vi "Scan Double.vi"(8 "error in (no error)":errorcluster, 11 "Scan Driver in":refnum<class "Scan Driver.lvclass">) -> (0 "error out":errorcluster, 2 "Again?":bool, 3 "Scan Driver out":refnum<class "Scan Driver.lvclass">)   [LabVIEW 2012, in "Scan Driver.lvclass"]
doc: "Main method for Scan Driver. Scan over the given Scanner, read data points from the given Readable, generate an onscreen graph, and write a data file."
uses:
  Scan Driver.lvclass
  File IO/File IO.lvclass
  Global/File Locations.vi
  Global/Flags.vi
  Global/Misc.vi
  Scan Graph.ctl
  Scanners/Scanner/Scanner.lvclass
  Readers/Reader/Reader.lvclass
  Scanners/Double Scanner/Double Scanner.lvclass
  Instruments/Utility Classes/Readable/X.ctl
  Instruments/Utility Classes/Readable/Readable.lvclass
panel:
  out "Data Monitor 2D":T2(array[cluster])
  out "?":string
  out "progress":string
  out "Time Estimate":string
  out "date":timestamp
  out "timedisp":string
  in  "log?":bool
  out "cpshigh":dbl caption="CPS High"
  in  "restart":bool
  out "busybar":bool[](array[boolean])
  out "done?":bool caption="Done"
  in  "Exit":bool
  in  "stop":bool
  in  "?":bool
  out "Primary Graph":T3(graph) caption="cpsgraph"
  out "time":dbl
  out "Secondary Graph":T3(graph)
  # "Log"
  # "Linear"
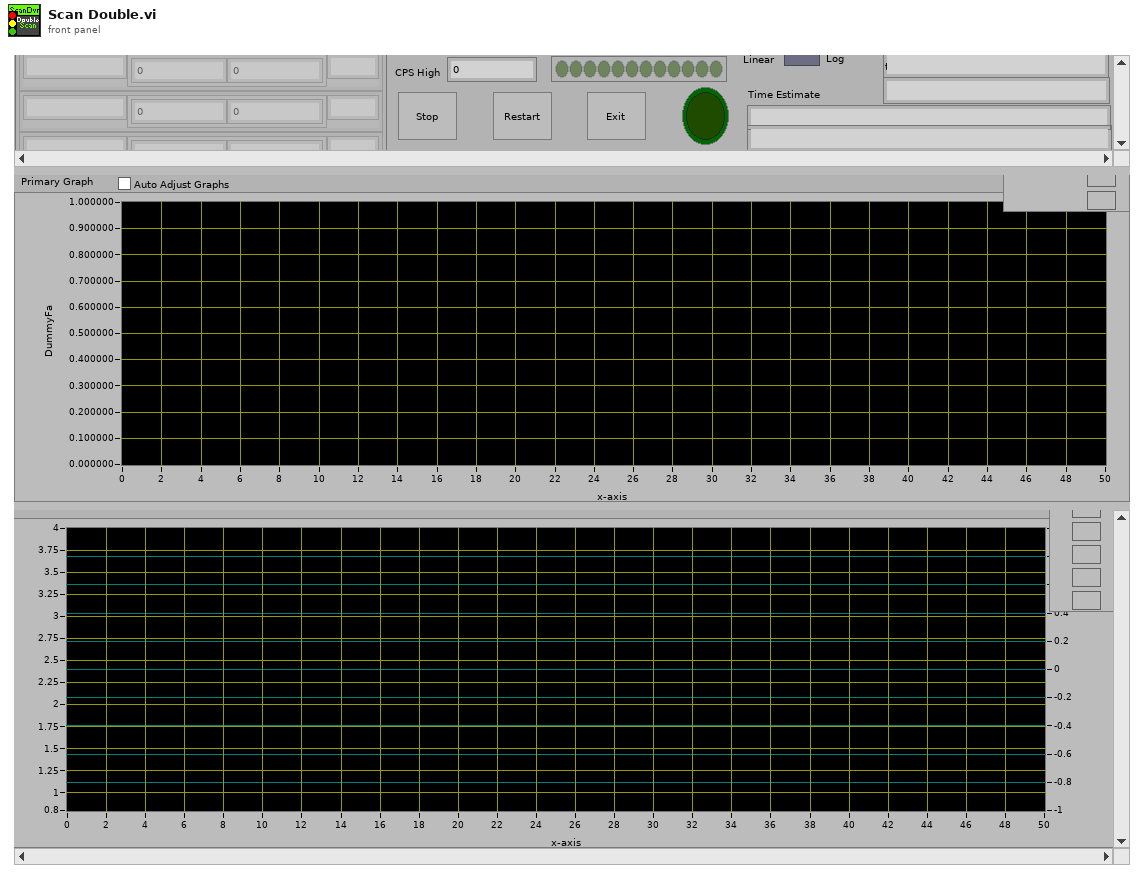
[diagram p1: front panel]
types:
  T1 = typedef "Readable.lvclass/X.ctl" = dbl
  T2 = cluster{"Name":string, "Array":T1[], "Unit":string}[]
  T3 = typedef "Scan Driver.lvclass/Scan Graph.ctl" = cluster{"point array":cluster{"x":dbl, "y":dbl}[]}[]
  T4 = typedef "Scanner.lvclass/Range.ctl" = cluster{"xi":dbl, "xf":dbl, "dx":dbl, "Return to...?":bool, "Return to":dbl}
  T5 = typedef "Readable.lvclass/Data Channels.ctl" = T6[]
  T6 = typedef "Readable.lvclass/Data Channel.ctl" = cluster{"Name":string, "Data Point":T7, "Unit":string}
  T7 = typedef "Readable.lvclass/Data Point.ctl" = cluster{"t":T8, "x":T1}
  T8 = typedef "Readable.lvclass/Time.ctl" = timestamp
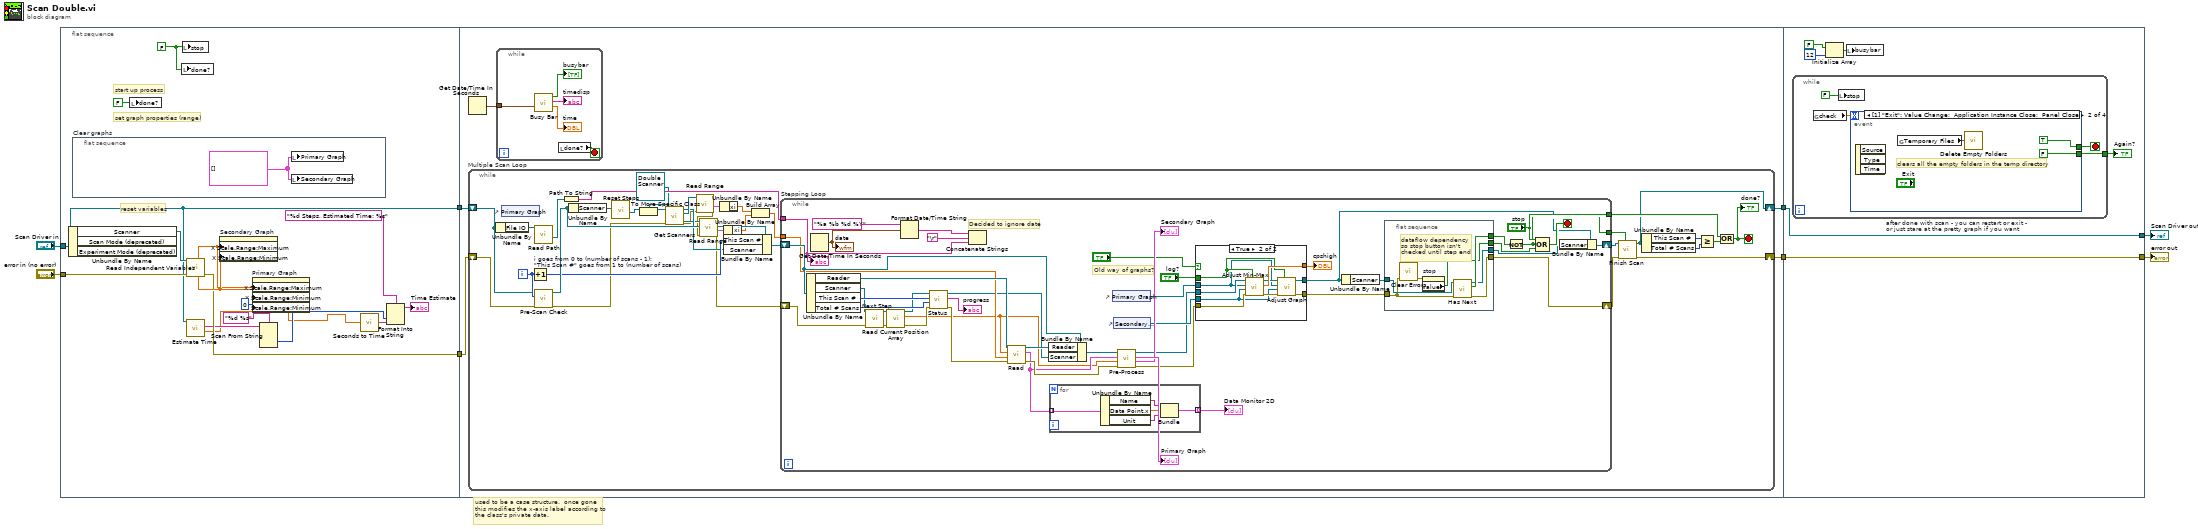
[diagram p0: block diagram]
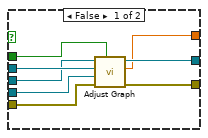
[diagram p2: hidden frame]
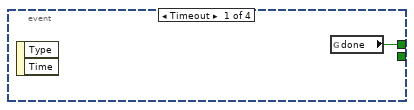
[diagram p3: hidden frame]
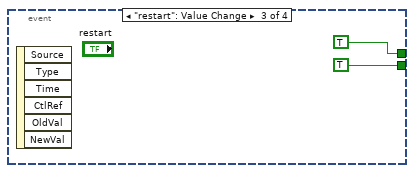
[diagram p4: hidden frame]
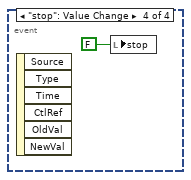
[diagram p5: hidden frame]
diagram:
  # "used to be a case structure.  once gone\nthis modifies the x-axis label according to\nthe class's private data."
  n1 = flat-sequence {
    tunnel: [w17] -> w4
    tunnel: [w21] -> w3
    tunnel: "error in (no error)" -> [w20]
    tunnel: "Scan Driver in" -> [w17]
    tunnel: w4 -> [w29]
    tunnel: [w28] -> w2
    tunnel: w3 -> [w27]
    tunnel: [w26] -> w1
    tunnel: [w147] -> w8
    tunnel: [w146] -> w5
    tunnel: w2 -> [w147]
    tunnel: w1 -> [w146]
    frame #0 {
      w19 = FALSE
      # "reset variables"
      # "start up process"
      # "set graph properties (range)"
      n2 = Unbundle By Name(w17) -> ("Scanner"=w18:refnum<class "Scanner.lvclass">)  [unwired: 2 out]
      n3 = flat-sequence "Clear graphs" {
        frame #0 {
          w25 = T3 []
          n4 = local write "Primary Graph"(w25) -> ()
          n5 = local write "Secondary Graph"(w25) -> ()
        }
      }
      n6 = local write "done?"(FALSE) -> ()
      n7 = local write "done?"(w19) -> ()
      n8 = local write "stop"(w19) -> ()
      n9 = call-dynamic "Read Independent Variables.vi"("error in (no error)"=w20, "Scanner.lvclass in"=w18) -> ("error out"=w21:errorcluster, "min value"=w24:dbl, "max value"=w23:dbl)  [unwired: 7 out]
      n10 = call "Estimate Time.vi"("Scan Driver in"=w17) -> ("Seconds"=w9:dbl[unit], "Time Estimate"=w15:string)  [unwired: 1 in, 8 out]
      n11 = property on="Secondary Graph" class="XYGraph (strict)"("X Scale.Range:Maximum"=w23, "X Scale.Range:Minimum"=w24) -> ()  [unwired: 2 in, 2 out]
      n12 = property on="Primary Graph" class="XYGraph (strict)"("X Scale.Range:Maximum"=w23, "X Scale.Range:Minimum"=w24, "Y Scale.Range:Minimum"=0) -> ()  [unwired: 2 in, 2 out]
      n13 = Scan From String(format string="%d %s", input string=w15) -> (output 1=w12:i32)  [unwired: 5 in, 3 out]
      n14 = call "Seconds to Time.vi"("Seconds"=w9) -> ("Time"=w11:string)
      n15 = Format Into String(format string="%d Steps, Estimated Time: %s", w12, w11) -> (resulting string=→"Time Estimate":string)  [unwired: 2 in, 1 out]
    }
    frame #1 {
      n16 = Get Date/Time In Seconds() -> (seconds since 1Jan1904=w30:timestamp)
      n17 = while "Multiple Scan Loop" {
        shift-right: [w61] -> w28
        shift-left: w29 -> [w54]
        shift-right: [w64] -> w26
        shift-left: w27 -> [w60]
        i -> [w55]
        stop <- w68 stop-if-true
        n18 = Unbundle By Name(w54) -> ("File IO"=w53:refnum<class "File IO.lvclass">)
        n19 = control-ref of="Primary Graph"() -> ()  [unwired: 1 out]
        n20 = Increment "i goes from 0 to (number of scans - 1);\n\"This Scan #\" goes from 1 to (number of scans)"(x=w55) -> (x+1=w56:i32)
        n21 = call-dynamic "Read Path.vi"("File IO.lvclass in"=w53) -> ("File Path"=w52:path)  [unwired: 6 in, 4 out]
        n22 = call "Pre-Scan Check.vi"("error in (no error)"=w60, "Current scan #"=w55, "Scan Driver in"=w54) -> ("error out"=w39:errorcluster, "Scan Driver out"=w57:refnum<class "Scan Driver.lvclass">)  [unwired: 2 in, 5 out]
        n23 = Path To String(path=w52) -> (string=w51:string)
        n24 = Unbundle By Name(w57) -> ("Scanner"=w59:refnum<class "Scanner.lvclass">)
        n25 = call "Reset Steps.vi"("Scanner.lvclass"=w59) -> ("Scanner.lvclass"=w47:refnum<class "Scanner.lvclass">)  [unwired: 10 in]
        n26 = To More Specific Class(target class=refnum<class "Double Scanner.lvclass"> refnum ("Double Scanner.lvclass"), reference=w47) -> (specific class reference=w46:refnum<class "Double Scanner.lvclass">)  [unwired: 1 in, 1 out]
        n27 = call-dynamic "Get Scanners.vi"("error in (no error)"=w39, "Double Scanner in"=w46) -> ("error out"=w38:errorcluster, "Scanner 2 out"=w42:refnum<class "Scanner.lvclass">, "Scanner 1 out"=w45:refnum<class "Scanner.lvclass">, "Double Scanner out"=w44:refnum<class "Double Scanner.lvclass">)  [unwired: 6 in]
        n28 = call-dynamic "Read Range.vi"("error in (no error)"=w38, "Scanner.lvclass in"=w45) -> ("error out"=w37:errorcluster, "Range"=w50:T4)  [unwired: 8 out]
        n29 = call-dynamic "Read Range.vi"("error in (no error)"=w37, "Scanner.lvclass in"=w42) -> ("error out"=w36:errorcluster, "Range"=w43:T4)  [unwired: 8 out]
        n30 = Unbundle By Name(w50) -> ("xi"=w40:dbl)
        n31 = Unbundle By Name(w43) -> ("xi"=w41:dbl)
        n32 = Bundle By Name(cluster=w57, "This Scan #"=w56, "Scanner"=w44) -> (w58:refnum<class "Scan Driver.lvclass">)
        n33 = Build Array(w40, w41) -> (w49:dbl[])
        n34 = while "Stepping Loop" {
          tunnel: ["stop"] -> w70
          shift-right: [w101] -> w65
          shift-left: w58 -> [w98]
          shift-right: [w104] -> w66
          shift-left: w36 -> [w100]
          tunnel: [w107] -> w63
          tunnel: w49 -> [w95]
          tunnel: w51 -> [w77]
          stop <- w115 stop-if-true
          # "Old way of graphs?"
          # "Decided to ignore date"
          n35 = Unbundle By Name(w98) -> ("Reader"=w97:refnum<class "Reader.lvclass">, "Scanner"=w99:refnum<class "Scanner.lvclass">, "This Scan #"=w106:u32, "Total # Scans"=w109:u32)
          n36 = Get Date/Time In Seconds() -> (seconds since 1Jan1904=w91:timestamp)
          "date" <- w91
          n37 = call-dynamic "Next Step.vi"("error in (no error)"=w100, "Scanner in"=w99) -> ("error out"=w74:errorcluster, "Scanner out"=w75:refnum<class "Scanner.lvclass">)  [unwired: 8 out]
          n38 = call-dynamic "Read Current Position Array.vi"("error in (no error)"=w74, "Scanner in"=w75) -> ("error out"=w73:errorcluster, "Position array"=w72:dbl[], "Scanner out"=w71:refnum<class "Scanner.lvclass">)  [unwired: 7 in]
          n39 = Format Date/Time String(time format string (%c)="%a %b %d %Y", seconds (now)=w91) -> (date/time string=w89:string)  [unwired: 1 in]
          n40 = call-dynamic "Status.vi"("error in (no error)"=w73, "totalscans"=w109, "scan#"=w106, "Scanner.lvclass in"=w71) -> ("error out"=w96:errorcluster, "scanprogress"=→"progress":string, "Scanner.lvclass out"=w87:refnum<class "Scanner.lvclass">)  [unwired: 5 out]
          n41 = Concatenate Strings(w89, "\r", w77) -> ()  [unwired: 1 out]
          n42 = call-dynamic "Read.vi"("error in (no error)"=w96, "Starting independent variables"=w95, "Current independent variables"=w72, "Reader in"=w97) -> ("error out"=w111:errorcluster, "Data Channels"=w93:T5, "Reader out"=w94:refnum<class "Reader.lvclass">)  [unwired: 5 out]
          n43 = Bundle By Name(cluster=w98, "Reader"=w94, "Scanner"=w87) -> (w110:refnum<class "Scan Driver.lvclass">)
          n44 = for {
            tunnel: w93 -> [w145] mode=indexing
            tunnel: [w141] -> w76 mode=indexing
            n45 = Unbundle By Name(w145) -> ("Name"=w142:string, "Data Point.x"=w143:T1, "Unit"=w144:string)
            n46 = Bundle("Name"=w142, "x"=w143, "Unit"=w144) -> (w141:cluster{"Name":string, "x":T1, "Unit":string})  [unwired: 1 in]
          }
          "Data Monitor 2D" <- w76
          n47 = control-ref of="Primary Graph"() -> (w86:refnum<vi>)
          n48 = control-ref of="Secondary Graph"() -> (w85:refnum<vi>)
          n49 = call "Pre-Process.vi"("error in"=w111, "Actual X Positions"=w72, "New Data Points"=w93, "Scan Driver.lvclass in"=w110) -> ("error out"=w83:errorcluster, "Secondary Graph"=→"Secondary Graph":T3, "Primary Graph"=→"Primary Graph":T3, "Scan Driver.lvclass out"=w84:refnum<class "Scan Driver.lvclass">)  [unwired: 3 in, 1 out]
          n50 = case shown="True" "?" {
            tunnel: w86 -> [w123 w125]
            tunnel: w85 -> [w122 w124]
            tunnel: w84 -> [w121 w133]
            tunnel: w83 -> [w120 w132]
            tunnel: [w116 w129] -> w82
            tunnel: [w118 w130] -> w81
            tunnel: [w117 w131] -> w80
            tunnel: "log?" -> [w119 w126]
            frame False {
              n51 = call "Adjust Graph.vi"("log?"=w119, "error in (no error)"=w120, "Secondary Graph"=w122, "Primary Graph"=w123, "Scan Driver.lvclass"=w121) -> ("error out"=w116:errorcluster, "High"=w117:dbl, "Scan Driver.lvclass out"=w118:refnum<class "Scan Driver.lvclass">)  [unwired: 4 in]
            }
            frame True {
              n52 = call "Adjust Min-Max.vi"("log?"=w126, "error in (no error)"=w132, "Secondary Graph"=w124, "Primary Graph"=w125, "Scan Driver.lvclass"=w133) -> ("error out"=w128:errorcluster, "High"=w131:dbl, "Scan Driver.lvclass out"=w127:refnum<class "Scan Driver.lvclass">)  [unwired: 3 in, 1 out]
              n53 = call "Adjust Graph.vi"("log?"=w126, "error in (no error)"=w128, "Secondary Graph"=w124, "Primary Graph"=w125, "Scan Driver.lvclass"=w127) -> ("error out"=w129:errorcluster, "Scan Driver.lvclass out"=w130:refnum<class "Scan Driver.lvclass">)  [unwired: 4 in, 1 out]
            }
          }
          "cpshigh" <- w80
          n54 = Unbundle By Name(w81) -> ("Scanner"=w103:refnum<class "Scanner.lvclass">)
          n55 = flat-sequence {
            tunnel: [w140] -> w105
            tunnel: w82 -> [w135]
            tunnel: [w139] -> w104
            tunnel: w103 -> [w138]
            tunnel: [w137] -> w102
            tunnel: [w134] -> w92
            frame #0 {
              # "dataflow dependency\nso stop button isn't\nchecked until step end"
              n56 = call <vilib>:"Clear Errors.vi"("error in (no error)"=w135) -> ("error out"=w136:errorcluster)  [unwired: 6 in]
              n57 = property on="stop" class="Bool (strict)"(error in=w136) -> ("Value"=w134:bool)  [unwired: 1 in, 2 out]
              n58 = call-dynamic "Has Next.vi"("error in (no error)"=w135, "Scanner.lvclass in"=w138) -> ("error out"=w139:errorcluster, "Again?"=w140:bool, "Scanner.lvclass out"=w137:refnum<class "Scanner.lvclass">)  [unwired: 7 out]
            }
          }
          n59 = Not(x=w105) -> (.not. x?=w107:bool)
          n60 = Compound Arithmetic op=OR("stop", w107, w92) -> (w115:bool)
          n61 = Bundle By Name(cluster=w81, "Scanner"=w102) -> (w101:refnum<class "Scan Driver.lvclass">)
          "?" <- w77
        }
        n62 = call "Finish Scan.vi"("Scan finished successfully?"=w63, "error in"=w66, "Scan Driver.lvclass in"=w65) -> ("error out"=w64:errorcluster, "Scan Driver.lvclass out"=w61:refnum<class "Scan Driver.lvclass">)  [unwired: 2 in, 5 out]
        n63 = Unbundle By Name(w61) -> ("This Scan #"=w62:u32, "Total # Scans"=w67:u32)
        n64 = Greater Or Equal?(x=w62, y=w67) -> (x >= y?=w69:bool)
        n65 = Compound Arithmetic op=OR(w70, w69) -> (w68:bool)
        "done?" <- w68
      }
      n66 = while {
        tunnel: w30 -> [w34]
        stop <- w33 stop-if-true
        n67 = call "Busy Bar.vi"("basetime"=w34) -> ("Elapsed Seconds"=→"time":dbl, "Time"=→"timedisp":string, "Busy Bar"=→"busybar":bool[])  [unwired: 1 in, 7 out]
        n68 = local read "done?"() -> (w33:bool)
      }
    }
    frame #2 {
      n69 = while "after done with scan - you can restart or exit - or just stare at the pretty graph if you want" {
        tunnel: [w153] -> w148
        stop <- w152 stop-if-true
        n70 = global read "Misc.vi" "check"() -> (w154:dbl)
        n71 = local write "stop"(FALSE ("stop")) -> ()
        n72 = event shown="[1] \"Exit\": Value Change;  Application Instance Close;  Panel Close" {
          selector: _ -> [_ _ _ _]
          dyn-events: _ -> [_ _ _ _]
          timeout: w154 -> [_ _ _ _]
          tunnel: [w156 TRUE TRUE ("done") _] -> w152
          tunnel: [_ FALSE TRUE ("done") _] -> w153
          event Timeout {
            n73 = event-data() -> ()  [unwired: 3 out]
            n74 = global read "Flags.vi" "done"() -> (w156:bool)
          }
          event "Exit": Value Change; Application Instance Close; Panel Close {
            # "clears all the empty folders in the temp directory"
            n75 = event-data() -> ()  [unwired: 4 out]
            n76 = global read "File Locations.vi" "Temporary Files"() -> (w158:path)
            n77 = call "Delete Empty Folders.vi"("dirpath"=w158) -> ()  [unwired: 5 out]
          }
          event "restart": Value Change {
            n78 = event-data() -> ()  [unwired: 7 out]
          }
          event "stop": Value Change {
            n79 = event-data() -> ()  [unwired: 7 out]
            n80 = local write "stop"(FALSE) -> ()
          }
        }
      }
      "Again?" <- w148
      n81 = Initialize Array(FALSE, 12) -> (w151:bool[])
      n82 = local write "busybar"(w151) -> ()
    }
  }
  "Scan Driver out" <- w8
  "error out" <- w5
